vi "Calculate Next Index.vi"(10 "message":T1={"name"="", "message type"="BC to RT", "endpoint Tx"={"terminal address"=0, "subaddress"=0}, "endpoint Rx"={"terminal address"=0, "subaddress"=0}, "create timestamp channel"=FALSE, "mode code"=0, "number of words"=0, "parameters"=[]}, 11 "index":i32) -> (3 "next index":i32)   [LabVIEW 2023, in "Ballard MIL-STD-1553 Engine Support.lvlib" / "Custom Device.lvlib"]
uses:
  Custom Device.lvlib
  Shared/Message Definition.ctl
  Shared/Message Type.ctl
  Shared/Terminal Endpoint.ctl
  Shared/Address.ctl
  Shared/Parameter Definition.ctl
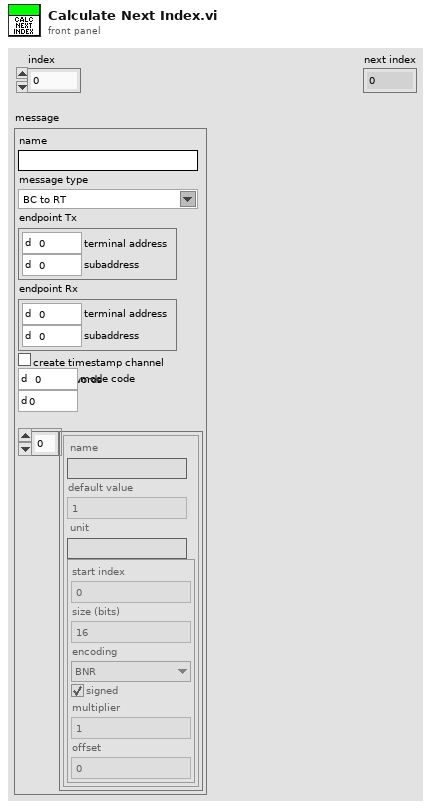
[diagram p1: front panel]
types:
  T1 = typedef "Message Definition.ctl" = cluster{"name":string, "message type":T2, "endpoint Tx":T3, "endpoint Rx":T3, "create timestamp channel":bool, "mode code":u16, "number of words":u16, "parameters":cluster{"name":string, "default value":dbl, "unit":string, "parameter definition":T5}[]}
  T2 = typedef "Message Type.ctl" = string
  T3 = typedef "Terminal Endpoint.ctl" = cluster{"terminal address":T4, "subaddress":T4}
  T4 = typedef "Address.ctl" = u16
  T5 = typedef "Parameter Definition.ctl" = cluster{"start index":i32, "size (bits)":i32, "encoding":enum16{"BNR", "BCD", "Discrete"}, "signed":bool, "multiplier":dbl, "offset":dbl}
  T6 = cluster{"name":string, "default value":dbl, "unit":string, "parameter definition":T5}[]
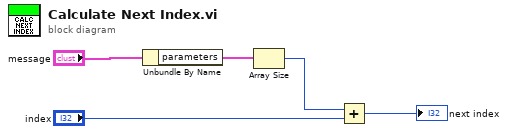
[diagram p0: block diagram]
diagram:
  n1 = Unbundle By Name("message") -> ("parameters"=w5:T6)
  n2 = Array Size(array=w5) -> (size(s)=w1:i32)
  n3 = Add(x=w1, y="index") -> (x+y=→"next index":i32)
